vi "Secondary Moniter.vi"() -> ()   [LabVIEW 2018]
uses:
  <vilib>/Rock Robotics/Network Tables/NT Read Number.vi
  <vilib>/Rock Robotics/Network Tables/NT Read Boolean.vi
panel:
  out "XY Graph":cluster{"Y":dbl[], "Y":dbl[]}[](graph)
  out "Low Gear":bool
  out "High Gear":bool
  out "Climber":bool
  out "Robot Centric":bool
  out "Field Centric":bool
  out "Tracks":bool caption="Brakes"
  out "Match Time":string
  out "Camera Image 2":T1(plugin-control)
  out "PSI":dbl(slide) scale=0.0..160.0
  out "Gyro":cluster{dbl, dbl}(knob) scale=0.0..360.0 scale format="%#.3g"
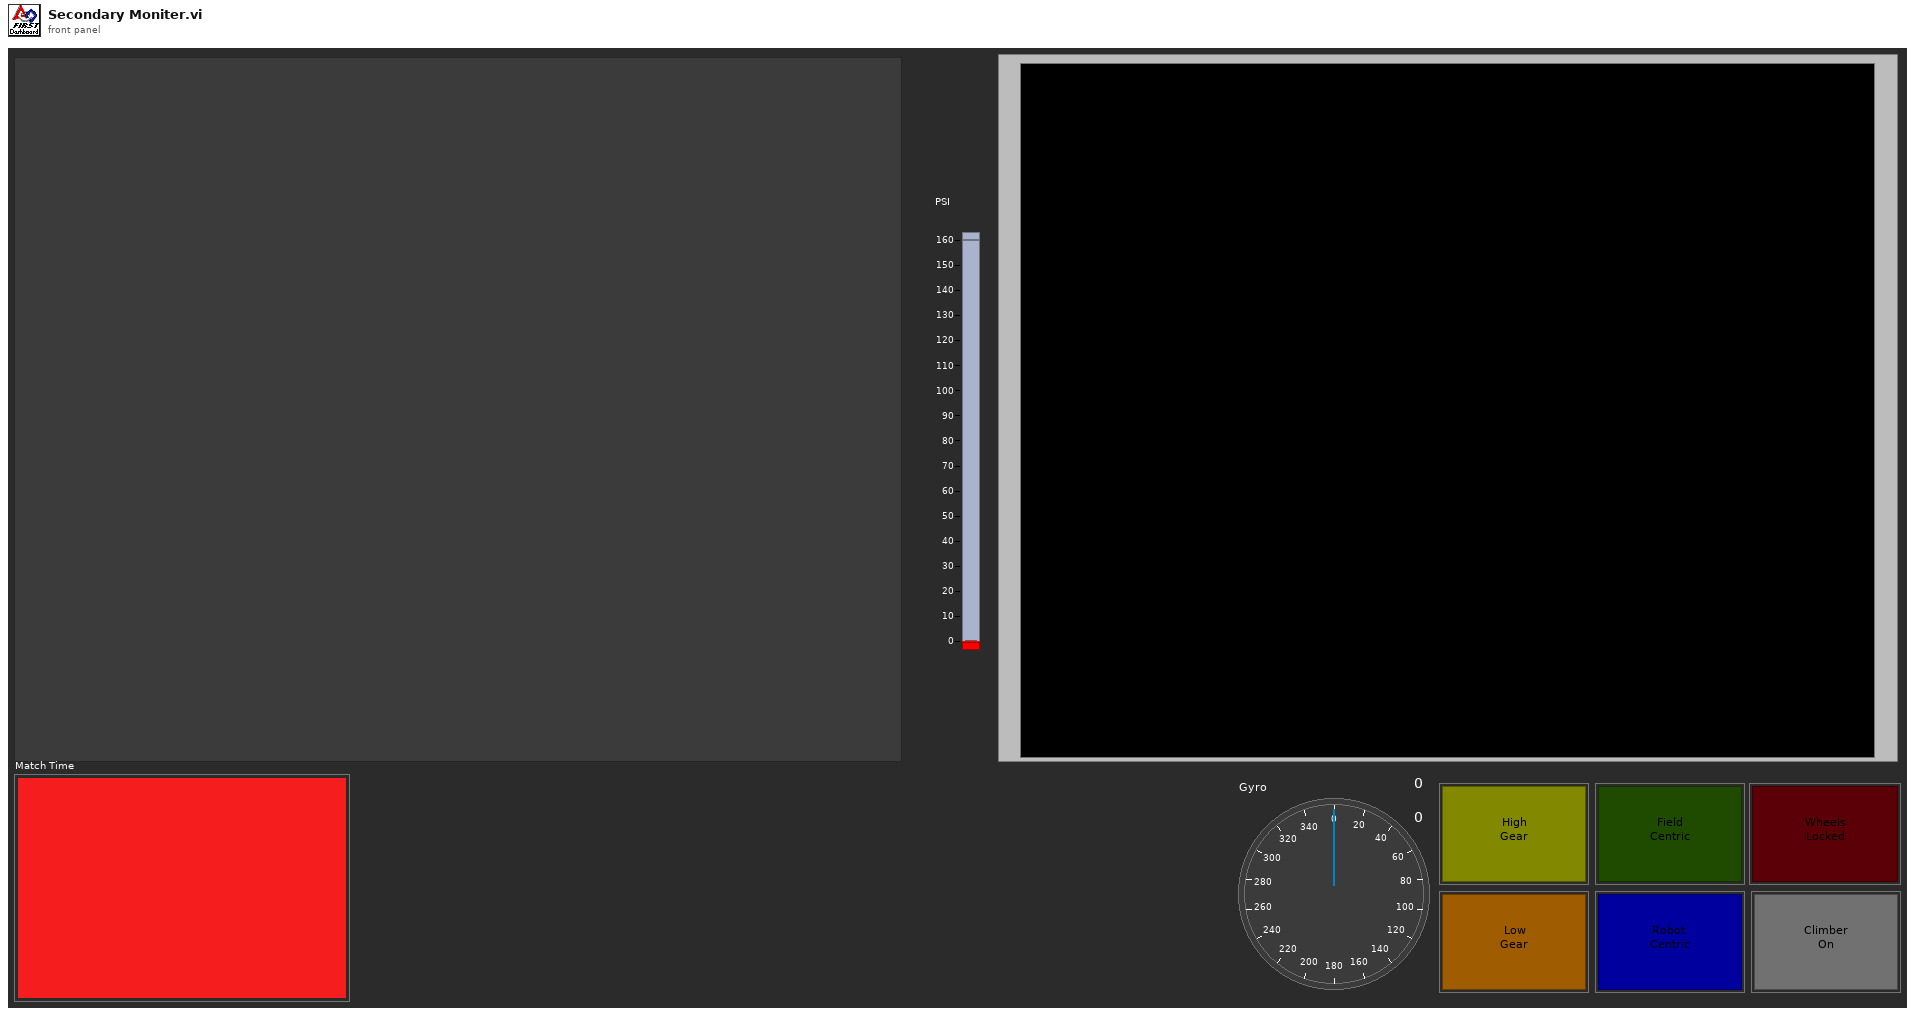
[diagram p1: front panel]
types:
  T1 = typedef "IMAQ Image.ctl" = refnum<image>
  T2 = typedef "LVDateTimeRec.ctl" = cluster{"fractional second":dbl, "second":i32, "minute":i32, "hour":i32, "day of month":i32, "month":i32, "year":i32, "day of week":i32, "day of year":i32, "DST":i32}
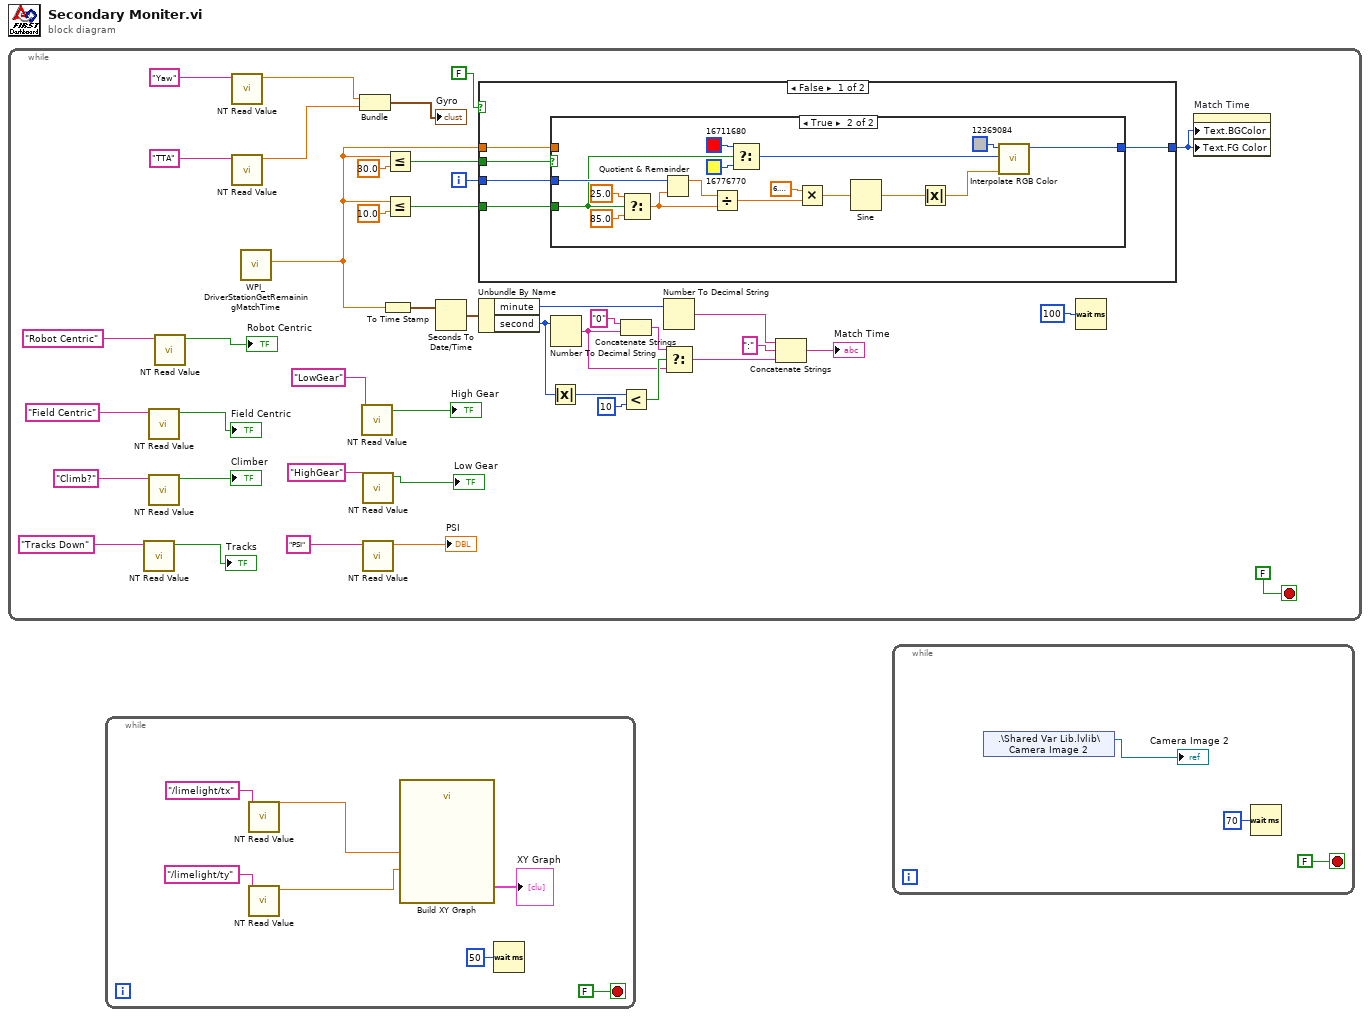
[diagram p0: block diagram]
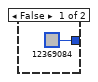
[diagram p2: hidden frame]
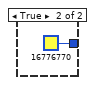
[diagram p3: hidden frame]
diagram:
  n1 = while {
    i -> [w21]
    stop <- FALSE stop-if-true
    n2 = call-poly <vilib>:"NT Read Value.vi"("Name"="Tracks Down") -> ("Boolean"=→"Tracks":bool)  [unwired: 9 in, 1 out]
    n3 = call-poly <vilib>:"NT Read Value.vi"("Name"="Field Centric") -> ("Boolean"=→"Field Centric":bool)  [unwired: 9 in, 1 out]
    n4 = call-poly <vilib>:"NT Read Value.vi"("Name"="Climb?") -> ("Boolean"=→"Climber":bool)  [unwired: 9 in, 1 out]
    n5 = call-poly <vilib>:"NT Read Value.vi"("Name"="Robot Centric") -> ("Boolean"=→"Robot Centric":bool)  [unwired: 9 in, 1 out]
    n6 = call-poly <vilib>:"NT Read Value.vi"("Name"="Yaw") -> ("Numeric"=w2:dbl)  [unwired: 9 in, 1 out]
    n7 = call-poly <vilib>:"NT Read Value.vi"("Name"="TTA") -> ("Numeric"=w3:dbl)  [unwired: 9 in, 1 out]
    n8 = call <vilib>:"WPI_DriverStationGetRemainingMatchTime.vi"() -> ("Match Time(s)"=w13:sgl)  [unwired: 10 in, 1 out]
    n9 = Bundle("Numeric"=w2, "Numeric"=w3) -> (→"Gyro":cluster{"Numeric":dbl, "Numeric":dbl})  [unwired: 1 in]
    n10 = call-poly <vilib>:"NT Read Value.vi"("Name"="LowGear") -> ("Boolean"=→"High Gear":bool)  [unwired: 9 in, 1 out]
    n11 = call-poly <vilib>:"NT Read Value.vi"("Name"="HighGear") -> ("Boolean"=→"Low Gear":bool)  [unwired: 9 in, 1 out]
    n12 = call-poly <vilib>:"NT Read Value.vi"("Name"="PSI") -> ("Numeric"=→"PSI":dbl)  [unwired: 9 in, 1 out]
    n13 = To Time Stamp(1:w13) -> (0:w22:timestamp)
    n14 = Less Or Equal?(x=w13, y=30.0) -> (x <= y?=w17:bool)
    n15 = Less Or Equal?(x=w13, y=10.0) -> (x <= y?=w18:bool)
    n16 = Seconds To Date/Time(time stamp (now)=w22) -> (date time rec=w15:T2)  [unwired: 1 in]
    n17 = case shown="False" FALSE {
      tunnel: w17 -> [w48 _]
      tunnel: w18 -> [w47 _]
      tunnel: [w46 u32 16776770 ("Color")] -> w16
      tunnel: w13 -> [w45 _]
      tunnel: w21 -> [w44 _]
      frame False {
        n18 = case shown="True" w48 {
          tunnel: w47 -> [_ w53]
          tunnel: [u32 12369084 ("Color") w54] -> w46
          tunnel: w45 -> [_ _]
          tunnel: w44 -> [_ w57]
          frame False {
          }
          frame True {
            n19 = Select(t=25.0, s=w53, f=85.0) -> (s? t:f=w50:dbl)
            n20 = Quotient & Remainder(x=w57, y=w50) -> (x-y*floor(x/y)=w60:dbl)  [unwired: 1 out]
            n21 = Divide(x=w60, y=w50) -> (x/y=w59:dbl)
            n22 = Select(t=u32 16711680 ("Color"), s=w53, f=u32 16776770 ("Color")) -> (s? t:f=w56:u32)
            n23 = Multiply(x=6.283185307179586, y=w59) -> (x*y=w62:dbl)
            n24 = Sine(x=w62) -> (sin(x)=w61:dbl)
            n25 = Absolute Value(x=w61) -> (abs(x)=w58:dbl)
            n26 = call "Interpolate RGB Color.vi"("Proportion"=w58, "Target Color"=w56, "Base Color"=u32 12369084 ("Color")) -> ("Result Color"=w54:u32)  [unwired: 8 in]
          }
        }
      }
      frame True {
      }
    }
    n27 = Unbundle By Name(w15) -> ("minute"=w23:i32, "second"=w24:i32)
    n28 = Absolute Value(x=w24) -> (abs(x)=w32:i32)
    n29 = Number To Decimal String(number=w24) -> (decimal integer string=w27:string)  [unwired: 1 in]
    n30 = Concatenate Strings("0" ("string"), w27) -> (w29:string)
    n31 = Less?(x=w32, y=10) -> (x < y?=w28:bool)
    n32 = Number To Decimal String(number=w23) -> (decimal integer string=w33:string)  [unwired: 1 in]
    n33 = Select(t=w29, s=w28, f=w27) -> (s? t:f=w26:string)
    n34 = Concatenate Strings(w33, ":" ("string"), w26) -> (→"Match Time":string)
    n35 = Wait (ms)(milliseconds to wait=u32 100) -> ()  [unwired: 1 out]
    n36 = property on="Match Time" class="Str"("Text.BGColor"=w16, "Text.FG Color"=w16) -> ()  [unwired: 2 in, 2 out]
  }
  n37 = while {
    stop <- FALSE stop-if-true
    n38 = call-poly <vilib>:"NT Read Value.vi"("Name"="/limelight/tx") -> ("Numeric"=w70:dbl)  [unwired: 9 in, 1 out]
    n39 = call-poly <vilib>:"NT Read Value.vi"("Name"="/limelight/ty") -> ("Numeric"=w69:dbl)  [unwired: 9 in, 1 out]
    n40 = call "Build XY Graph"("Y Input"=w69, "X Input"=w70) -> ("XY Graph"=→"XY Graph":cluster{"X":dbl[], "Y":dbl[]}[])  [unwired: 8 in, 1 out]
    n41 = Wait (ms)(milliseconds to wait=u32 50) -> ()  [unwired: 1 out]
  }
  n42 = while {
    stop <- FALSE stop-if-true
    n43 = shared-variable ".\\Shared Var Lib.lvlib\\Camera Image 2"() -> (→"Camera Image 2":refnum<image>)  [unwired: 1 in, 1 out]
    n44 = Wait (ms)(milliseconds to wait=u32 70) -> ()  [unwired: 1 out]
  }
